vi "getSubData_Device_MAGSpec_AllinOne.vi"(9 "variant in":variant, 10 "SubscriberCluster":T1, 11 "timeout":i32=3000) -> (1 "variant out":variant, 2 "OK":bool[](array[boolean]))   [LabVIEW 2011]
uses:
  SubscriberCluster_TypDEf.ctl
  tcp_new_data_event.ctl
  tcp new data cluster.ctl
  IMAQ Image.ctl
  NI_Vision_Development_Module.lvlib
panel:
  out "Devices 2":string[](array[string])
  out "userID":string
  out "timed out?":bool
  out "Devices ALL":string[](array[string])
  out "Devices":string[](array[string])
  out "element":string[][](array[string])
  out "Numeric":i32
  out "all lower case string":string[](array[string])
  out "timeout":bool
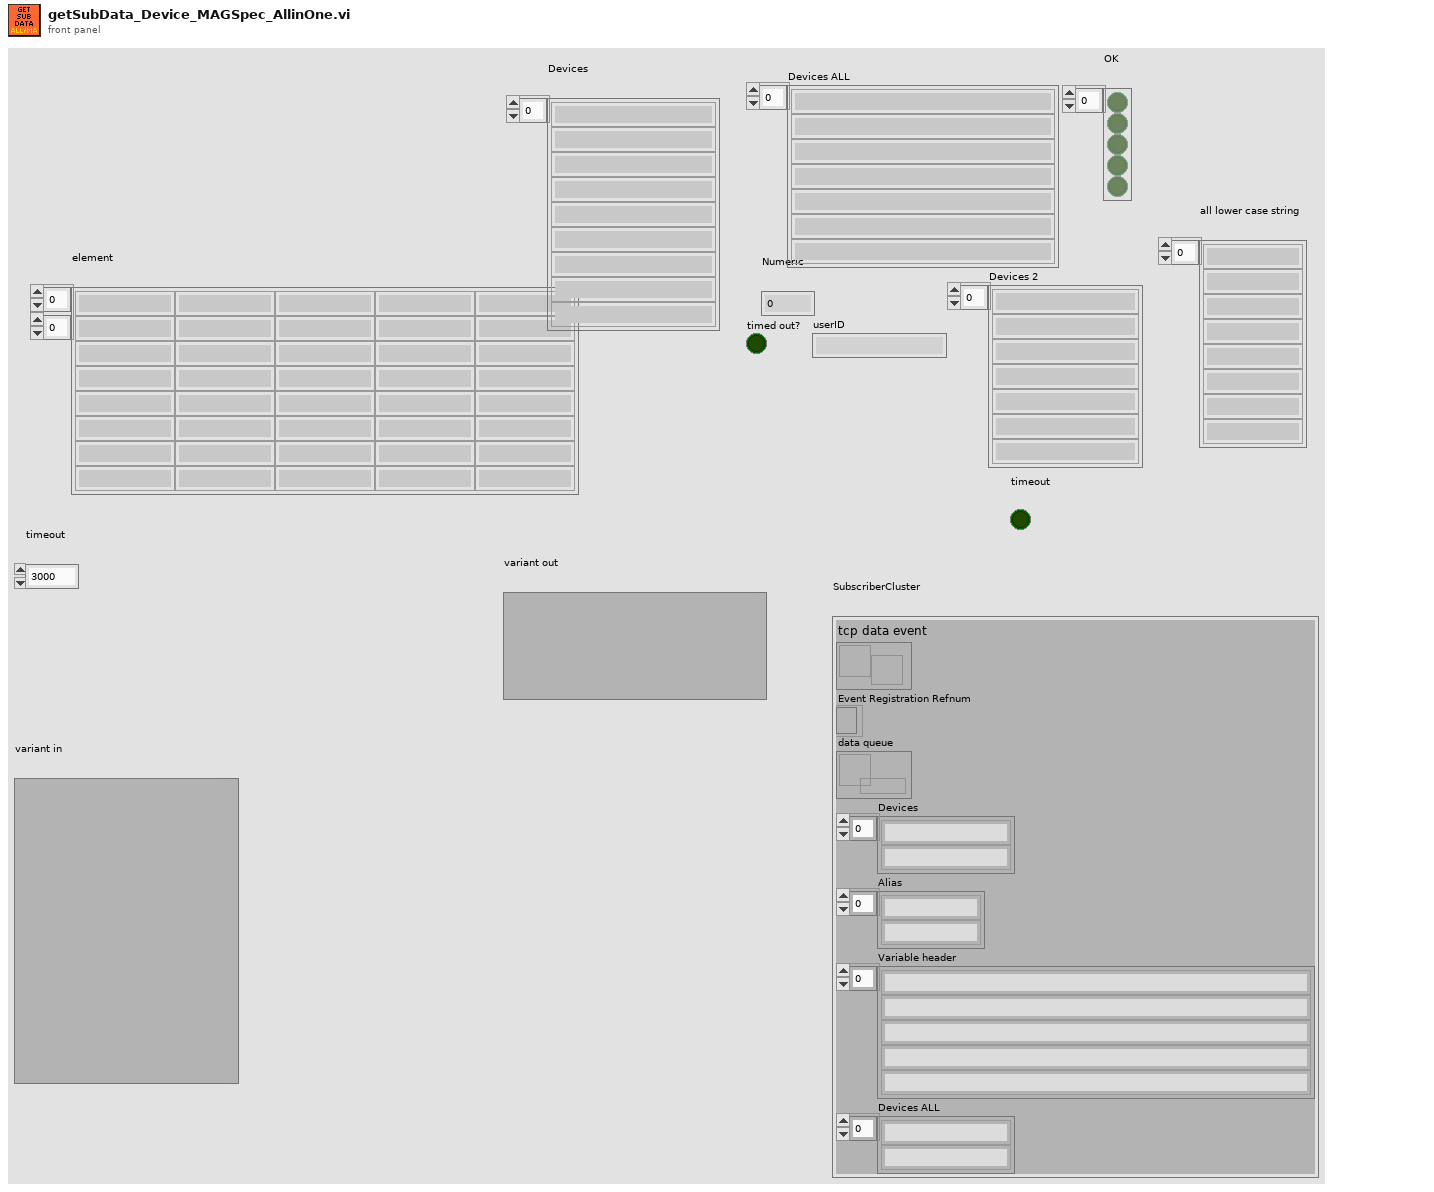
[diagram p1: front panel]
types:
  T1 = typedef "SubscriberCluster_TypDEf.ctl" = cluster{"tcp data event":T2, "Event Registration Refnum":refnum<event-registration>, "data queue":refnum<queue>, "Devices":string[], "Alias":string[], "Variable header":string[], "Devices ALL":string[]}
  T2 = typedef "tcp_new_data_event.ctl" = refnum<user-event>
  T3 = typedef "IMAQ Image.ctl" = refnum<image>
  T4 = typedef "Type Descriptor Enumeration__ogtk.ctl" = enum8{"<Null>", "I8", "I16", "I32", "I64", "U8", "U16", "U32", "U64", "SGL", "DBL", "EXT", "CSG", "CDB", "CXT", "0x0F", "0x10", "0x11", "0x12", "0x13", "0x14", "Enum U8", "Enum U16", "Enum U32", "Enum U64", "SGL PQ", "DBL PQ", "EXT PQ", "CSG PQ", "CDB PQ", "CXT PQ", "0x1F", "0x20", "Boolean", "0x22", "0x23", "0x24", "0x25", "0x26", "0x27", "0x28", "0x29", "0x2A", "0x2B", "0x2C", "0x2D", "0x2E", "0x2F", "String", "0x31", "Path", "Pict", "0x34", "0x35", "0x36", "DAQ", "0x38", "0x39", "0x3A", "0x3B", "0x3C", "0x3D", "0x3E", "0x3F", "Array", "0x41", "0x42", "0x43", "0x44", "0x45", "0x46", "0x47", "0x48", "0x49", "0x4A", "0x4B", "0x4C", "0x4D", "0x4E", "0x4F", "Cluster", "0x51", "0x52", "Variant", "Waveform", "0x55", "0x56", "0x57", "0x58", "0x59", "0x5A", "0x5B", "0x5C", "0x5D", "0x5E", "0x5F", "0x60", "0x61", "0x62", "0x63", "0x64", "0x65", "0x66", "0x67", "0x68", "0x69", "0x6A", "0x6B", "0x6C", "0x6D", "0x6E", "0x6F", "Refnum"}
  T5 = typedef "Image Type" = u32
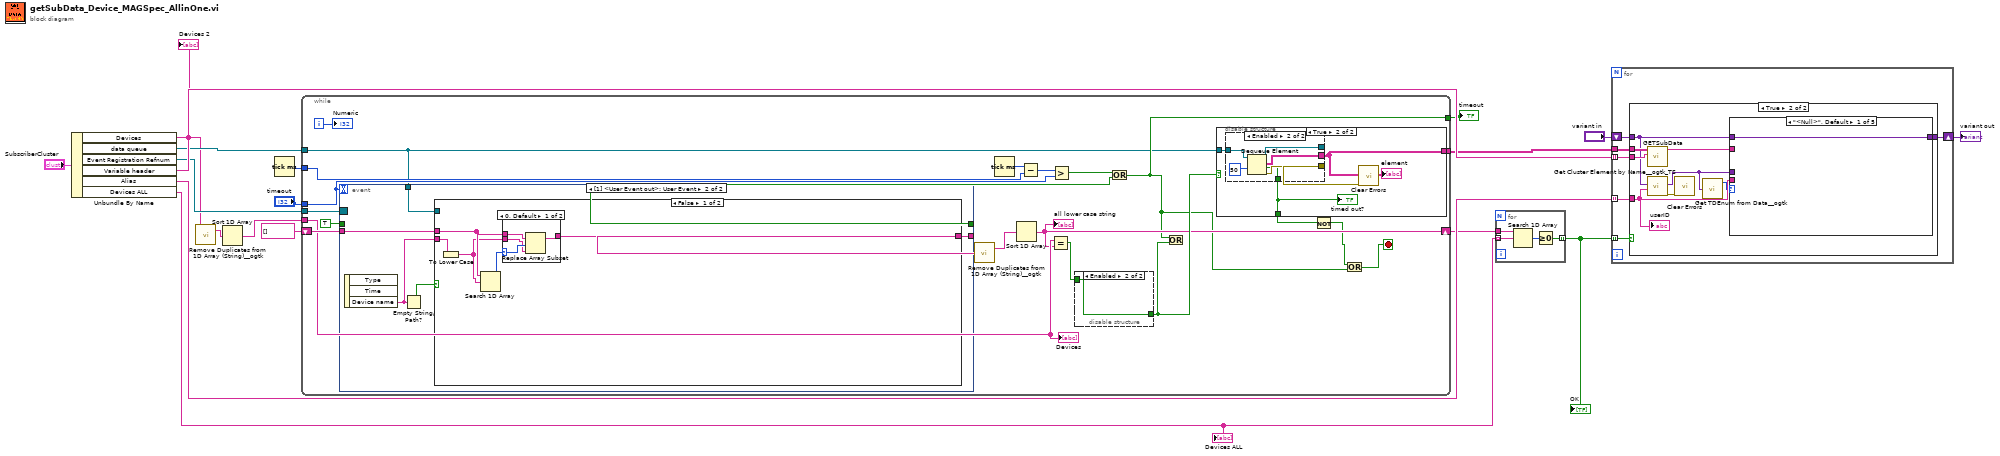
[diagram p0: block diagram]
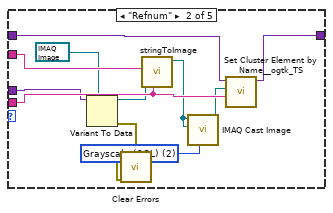
[diagram p3: hidden frame]
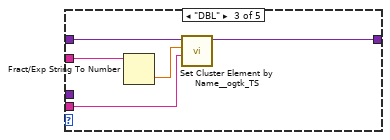
[diagram p4: hidden frame]
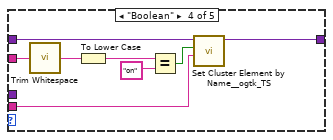
[diagram p5: hidden frame]
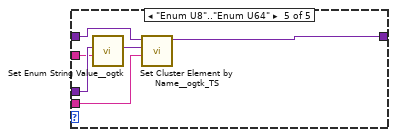
[diagram p6: hidden frame]
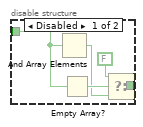
[diagram p7: hidden frame]
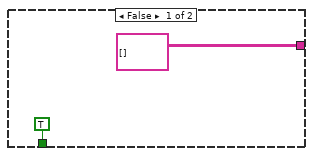
[diagram p8: hidden frame]
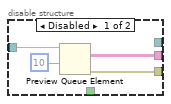
[diagram p9: hidden frame]
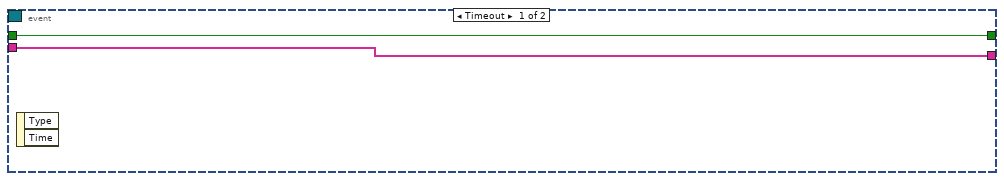
[diagram p10: hidden frame]
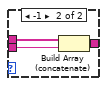
[diagram p11: hidden frame]
diagram:
  n1 = Unbundle By Name("SubscriberCluster") -> ("Devices"=w2:string[], "data queue"=w13:refnum<queue>, "Event Registration Refnum"=w12:refnum<event-registration>, "Variable header"=w14:string[], "Alias"=w9:string[], "Devices ALL"=w4:string[])
  "Devices ALL" <- w4
  "Devices 2" <- w2
  n2 = call "Remove Duplicates from 1D Array (String)__ogtk.vi"("Input Array"=w2) -> ("Output Array"=w1:string[])  [unwired: 1 out]
  n3 = Sort 1D Array(array=w1) -> (sorted array=w3:string[])
  n4 = Tick Count (ms)() -> (millisecond timer value=w7:u32)
  n5 = while {
    tunnel: w12 -> [w40]
    tunnel: w13 -> [w19]
    tunnel: [w30] -> w11
    shift-right: [w26] -> w6
    shift-left: string[] [] -> [w38]
    tunnel: w3 -> [w37]
    tunnel: "timeout" -> [w34]
    tunnel: [w21] -> w8
    tunnel: w7 -> [w36]
    i -> [w29]
    stop <- w20 stop-if-true
    n6 = event shown="[1] <User Event out>: User Event" {
      selector: w40 -> [_ _]
      dyn-events: _ -> [_ _]
      timeout: w34 -> [_ _]
      tunnel: [w64 _] -> w33
      tunnel: TRUE -> [w64 _]
      tunnel: [w63 w69] -> w25
      tunnel: w38 -> [w63 w66]
      tunnel: w19 -> [_ w65]
      event Timeout {
        n7 = event-data() -> ()  [unwired: 1 in, 2 out]
      }
      event User Event {
        n8 = event-data() -> ("Device name"=w68:string)  [unwired: 1 in, 2 out]
        n9 = Empty String/Path?(string/path=w68) -> (empty?=w67:bool)
        n10 = case shown="False" w67 {
          tunnel: w68 -> [w71 _]
          tunnel: [w74 w82] -> w69
          tunnel: w66 -> [w73 w82]
          tunnel: w65 -> [_ _]
          frame False {
            n11 = To Lower Case(string=w71) -> (all lower case string=w70:string)
            n12 = Search 1D Array(1D array=w73, element=w70) -> (index of element=w72:i32)  [unwired: 1 in]
            n13 = case shown="0, Default" w72 {
              selector: w72 -> [w76 _]
              tunnel: w70 -> [w75 w81]
              tunnel: [w77 w80] -> w74
              tunnel: w73 -> [w78 w79]
              frame 0, Default {
                n14 = Replace Array Subset(array=w78, new element=w75, index=w76) -> (w77:string[])
              }
              frame -1 {
                n15 = Build Array (concatenate)(w79, w81) -> (w80:string[])
              }
            }
          }
          frame True {
          }
        }
      }
    }
    n16 = call "Remove Duplicates from 1D Array (String)__ogtk.vi"("Input Array"=w25) -> ("Output Array"=w24:string[])  [unwired: 1 out]
    n17 = Tick Count (ms)() -> (millisecond timer value=w31:u32)
    n18 = Sort 1D Array(array=w24) -> (sorted array=w26:string[])
    "all lower case string" <- w26
    n19 = Subtract(x=w31, y=w36) -> (x-y=w35:u32)
    n20 = Equal?(x=w37, y=w26) -> (x = y?=w28:bool)
    n21 = Greater?(x=w35, y=w34) -> (0:w32:bool)
    n22 = disable-structure shown="Enabled" {
      disable-tunnel: w28 -> [w45 w46]
      disable-tunnel: [w41 w46] -> w27
      frame Disabled {
        n23 = And Array Elements(Boolean array=w45) -> (logical AND=w42:bool)
        n24 = Empty Array?(array=w45) -> (empty?=w44:bool)
        n25 = Select(t=FALSE ("empty?"), s=w44, f=w42) -> (s? t:f=w41:bool)
      }
      frame Enabled {
      }
    }
    n26 = Or(x=w32, y=w33) -> (x .or. y?=w21:bool)
    n27 = Or(x=w21, y=w27) -> ()  [unwired: 1 out]
    n28 = case shown="True" w27 {
      tunnel: w19 -> [_ w52]
      tunnel: [string[][] [] ("Data in") w50] -> w30
      tunnel: [TRUE ("timed out?") w49] -> w23
      frame False {
      }
      frame True {
        n29 = disable-structure shown="Enabled" {
          disable-tunnel: w52 -> [w55 w62]
          disable-tunnel: [w54 w61] -> w50
          disable-tunnel: [w53 w60] -> w51
          disable-tunnel: [_ w58] -> _
          disable-tunnel: [_ w57] -> w49
          frame Disabled {
            n30 = Preview Queue Element(queue=w55, timeout in ms (-1)=10) -> (element=w54:string[][], error out=w53:errorcluster)  [unwired: 1 in, 2 out]
          }
          frame Enabled {
            n31 = Dequeue Element(queue=w62, timeout in ms (-1)=50) -> (queue out=w58:refnum<queue>, element=w61:string[][], timed out?=w57:bool, error out=w60:errorcluster)  [unwired: 1 in]
          }
        }
        "element" <- w50
        "timed out?" <- w49
        n32 = call "Clear Errors.vi"("error in (no error)"=w51) -> ()  [unwired: 6 in, 1 out]
      }
    }
    n33 = Not(x=w23) -> (.not. x?=w22:bool)
    n34 = Or(x=w22, y=w21) -> (x .or. y?=w20:bool)
    "Numeric" <- w29
    "Devices" <- w37
  }
  "timeout" <- w8
  n35 = for {
    tunnel: w4 -> [w85] mode=indexing
    tunnel: w6 -> [w86]
    tunnel: [w83] -> w5 mode=indexing
    n36 = Search 1D Array(1D array=w86, element=w85) -> (index of element=w84:i32)  [unwired: 1 in]
    n37 = Greater Or Equal To 0?(x=w84) -> (x >= 0?=w83:bool)
  }
  "OK" <- w5
  n38 = for {
    tunnel: w11 -> [w91]
    shift-right: [w92] -> w15
    shift-left: "variant in" -> [w89]
    tunnel: w14 -> [w90] mode=indexing
    tunnel: w9 -> [w88] mode=indexing
    tunnel: w5 -> [w87] mode=indexing
    n39 = case shown="True" w87 {
      tunnel: [w93 w102] -> w92
      tunnel: w91 -> [_ w101]
      tunnel: w90 -> [_ w100]
      tunnel: w89 -> [w93 w98]
      tunnel: w88 -> [_ w97]
      frame False {
      }
      frame True {
        n40 = call "GETSubData.vi"("Variable Header"=w100, "Data out"=w101) -> ("delimiter (Tab)"=w99:string)  [unwired: 9 in]
        n41 = call "Get Cluster Element by Name__ogtk_TS.vi"("Element Name"=w97, "Cluster"=w98) -> ("error out"=w94:errorcluster, "VElement"=w95:variant)  [unwired: 7 in, 1 out]
        n42 = call "Clear Errors.vi"("error in (no error)"=w94) -> ()  [unwired: 6 in, 1 out]
        n43 = call "Get TDEnum from Data__ogtk.vi"("Data"=w95) -> ("Type Descriptor Enumeration"=w96:T4)  [unwired: 4 in]
        n44 = case shown="\"<Null>\", Default" w96 {
          tunnel: [w103 w107 w117 w126 w128] -> w102
          tunnel: w99 -> [_ w114 w119 w124 w132]
          tunnel: w98 -> [w103 w108 w118 w127 w131]
          tunnel: w97 -> [_ w113 w115 w125 w130]
          tunnel: w95 -> [_ w112 _ _ w133]
          frame "<Null>", Default {
          }
          frame "Refnum" {
            w105 = T5 2 items=["Grayscale (U8)", "Grayscale (I16)", "Grayscale (SGL)", "Complex (CSG)", "RGB (U32)", "HSL (U32)", "RGB (U64)", "Grayscale (U16)"] ("Image Type")
            n45 = Variant To Data(type=T3 refnum ("Image"), Variant=w112) -> (data=w110:T3, error out=w109:errorcluster)  [unwired: 1 in]
            n46 = call "Clear Errors.vi"("error in (no error)"=w109) -> ()  [unwired: 6 in, 1 out]
            n47 = call "stringToImage.vi"("label text (image name)"=w113, "data out"=w114, "Refnum in"=w110) -> ("Refnum out"=w106:T3)  [unwired: 5 in, 3 out]
            n48 = call "IMAQ Cast Image"("Image Type"=w105, "Image Dst"=w106, "Image Src"=w106) -> ("Image Dst Out"=w104:T3)  [unwired: 7 in, 1 out]
            n49 = call "Set Cluster Element by Name__ogtk_TS.vi"("Element Name (\"\": New Element Data Name)"=w113, "New Element Value"=w104, "Cluster"=w108) -> ("VCluster out"=w107:variant)  [unwired: 6 in, 2 out]
          }
          frame "DBL" {
            n50 = Fract/Exp String To Number(string=w119) -> (number=w116:dbl)  [unwired: 3 in, 1 out]
            n51 = call "Set Cluster Element by Name__ogtk_TS.vi"("Element Name (\"\": New Element Data Name)"=w115, "New Element Value"=w116, "Cluster"=w118) -> ("VCluster out"=w117:variant)  [unwired: 6 in, 2 out]
          }
          frame "Boolean" {
            n52 = call "Trim Whitespace.vi"("string"=w124) -> ("trimmed string"=w123:string)  [unwired: 1 in]
            n53 = To Lower Case(string=w123) -> (all lower case string=w122:string)
            n54 = Equal?(x=w122, y="on" ("x")) -> (x = y?=w120:bool)
            n55 = call "Set Cluster Element by Name__ogtk_TS.vi"("Element Name (\"\": New Element Data Name)"=w125, "New Element Value"=w120, "Cluster"=w127) -> ("VCluster out"=w126:variant)  [unwired: 6 in, 2 out]
          }
          frame "Enum U8".."Enum U64" {
            n56 = call "Set Enum String Value__ogtk.vi"("String Value"=w132, "Default Enum Value"=w133) -> ("Enum"=w129:variant)  [unwired: 8 in, 1 out]
            n57 = call "Set Cluster Element by Name__ogtk_TS.vi"("Element Name (\"\": New Element Data Name)"=w130, "New Element Value"=w129, "Cluster"=w131) -> ("VCluster out"=w128:variant)  [unwired: 6 in, 2 out]
          }
        }
        "userID" <- w97
      }
    }
  }
  "variant out" <- w15
